vi "ForwardKinematics_4Omni.vi"(0 "w1":dbl, 1 "Robot Radius (m)":dbl, 2 "Wheel Radius (m)":dbl, 5 "w2":dbl, 7 "w3":dbl, 9 "w4":dbl, 11 "error in (no error)":errorcluster) -> (4 "Vx":dbl, 6 "Vy":dbl, 8 "Omega":dbl, 15 "error out":errorcluster)   [LabVIEW 2017]
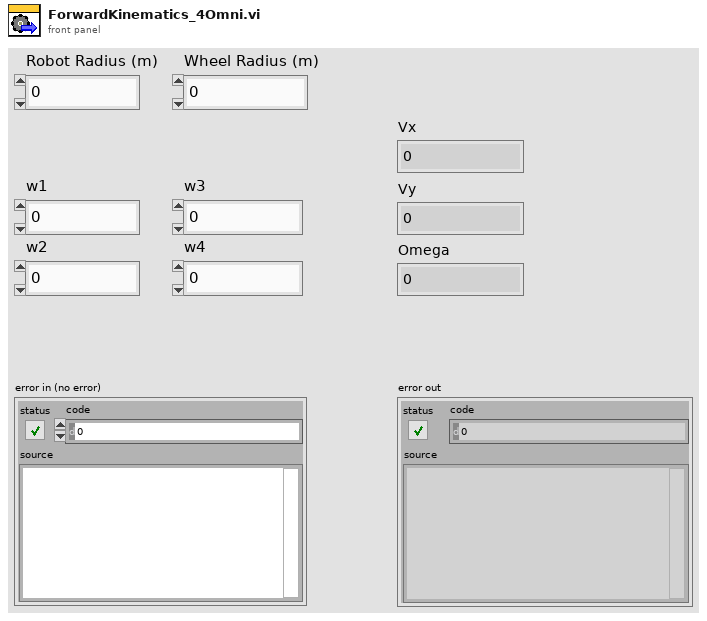
[diagram p1: front panel]
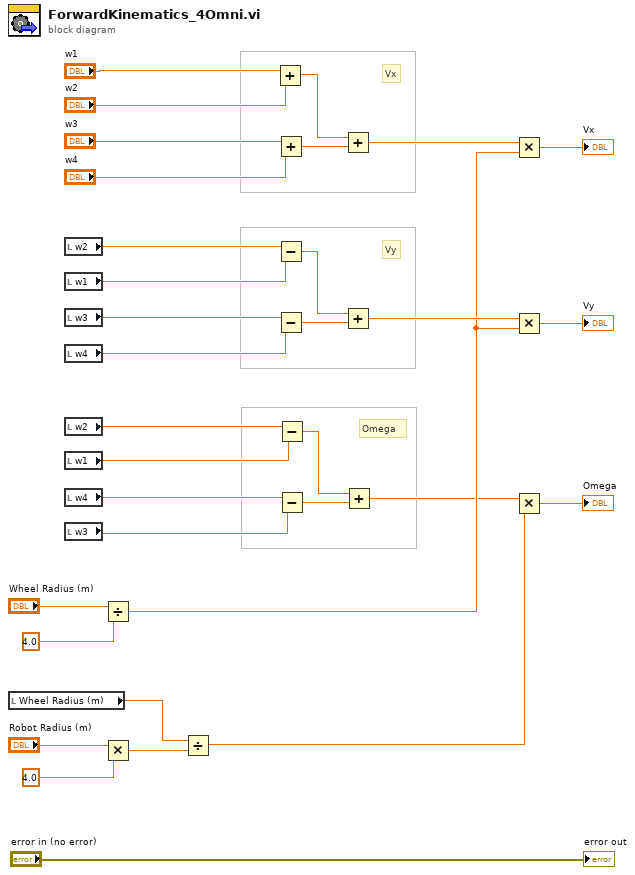
[diagram p0: block diagram]
diagram:
  # "Omega"
  # "Vy"
  # "Vx"
  n1 = local read "Wheel Radius (m)"() -> (w4:dbl)
  n2 = local read "w2"() -> (w21:dbl)
  n3 = local read "w1"() -> (w20:dbl)
  n4 = local read "w3"() -> (w18:dbl)
  n5 = local read "w4"() -> (w17:dbl)
  n6 = local read "w2"() -> (w10:dbl)
  n7 = local read "w1"() -> (w9:dbl)
  n8 = local read "w4"() -> (w8:dbl)
  n9 = local read "w3"() -> (w7:dbl)
  n10 = Divide(x="Wheel Radius (m)", y=4.0) -> (x/y=w13:dbl)
  n11 = Multiply(x="Robot Radius (m)", y=4.0) -> (x*y=w5:dbl)
  n12 = Divide(x=w4, y=w5) -> (x/y=w1:dbl)
  n13 = Add(x="w1", y="w2") -> (x+y=w25:dbl)
  n14 = Add(x="w3", y="w4") -> (x+y=w24:dbl)
  n15 = Subtract(x=w21, y=w20) -> (x-y=w19:dbl)
  n16 = Subtract(x=w18, y=w17) -> (x-y=w16:dbl)
  n17 = Subtract(x=w10, y=w9) -> (x-y=w12:dbl)
  n18 = Subtract(x=w8, y=w7) -> (x-y=w11:dbl)
  n19 = Add(x=w25, y=w24) -> (x+y=w23:dbl)
  n20 = Add(x=w19, y=w16) -> (x+y=w14:dbl)
  n21 = Add(x=w12, y=w11) -> (x+y=w2:dbl)
  n22 = Multiply(x=w23, y=w13) -> (x*y=→"Vx":dbl)
  n23 = Multiply(x=w14, y=w13) -> (x*y=→"Vy":dbl)
  n24 = Multiply(x=w2, y=w1) -> (x*y=→"Omega":dbl)
  "error out" <- "error in (no error)"
